vi "dictionary_to_units.vi"(8 "error in (no error)":errorcluster, 11 "data_set":variant) -> (0 "error out":errorcluster, 3 "units []":T1[](array[typedef]))   [LabVIEW 2015, in "lv-unit-conversion.lvlib"]
uses:
  lv-unit-conversion.lvlib
  public/_controls/unit.ctl
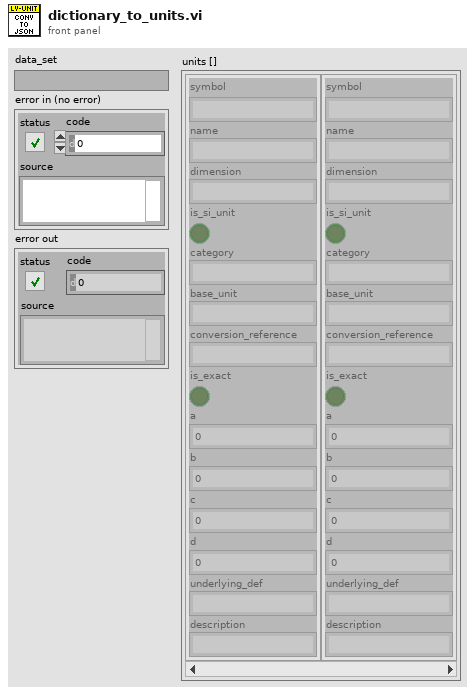
[diagram p1: front panel]
types:
  T1 = typedef "lv-unit-conversion.lvlib/unit.ctl" = cluster{"symbol":string, "name":string, "dimension":string, "is_si_unit":bool, "category":string, "base_unit":string, "conversion_reference":string, "is_exact":bool, "a":dbl, "b":dbl, "c":dbl, "d":dbl, "underlying_def":string, "description":string}
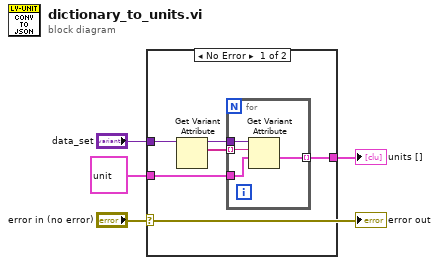
[diagram p0: block diagram]
diagram:
  n1 = case shown="No Error" "error in (no error)" {
    tunnel: "data_set" -> [w9 _]
    tunnel: [w6 _] -> w2
    tunnel: T1 {"symbol"="", "name"="", "dimension"="", "is_si_unit"=FALSE, "category"="", "base_unit"="", "conversion_reference"="", "is_exact"=FALSE, "a"=0.0, "b"=0.0, "c"=0.0, "d"=0.0, "underlying_def"="", "description"=""} ("unit_set") -> [w5 _]
    frame No Error {
      n2 = Get Variant Attribute(Variant=w9) -> (duplicate Variant=w7:variant, names=w8:string[])  [unwired: 3 in, 2 out]
      n3 = for {
        tunnel: w8 -> [w12] mode=indexing
        tunnel: w7 -> [w13]
        tunnel: w5 -> [w11]
        tunnel: [w10] -> w6 mode=indexing
        n4 = Get Variant Attribute(Variant=w13, name=w12, default value (empty Variant)=w11) -> (value=w10:T1)  [unwired: 1 in, 3 out]
      }
    }
    frame Error {
    }
  }
  "units []" <- w2
  "error out" <- "error in (no error)"
